vi "Equalizer.vi"() -> ()   [LabVIEW 2018]
uses:
  <vilib>/Analysis/2dsp.llb/Power Spectrum (DBL).vi
  <vilib>/Analysis/NI_AALPro.lvlib
panel:
  in  "False case signal":bool
  in  "Signal":dbl
  in  "Highpass":bool
  in  "Lowpass":bool
  in  "Bandpass":bool
  out "Highpass":bool
  out "Bandpass":bool
  out "Lowpass":bool
  out "Waveform Chart":dbl[](graph)
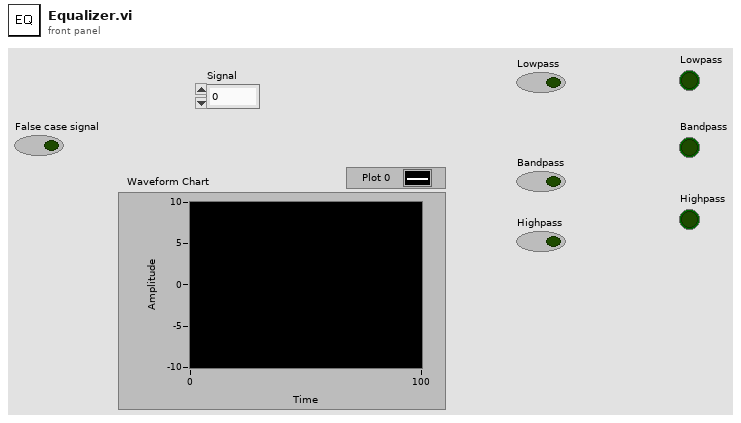
[diagram p1: front panel]
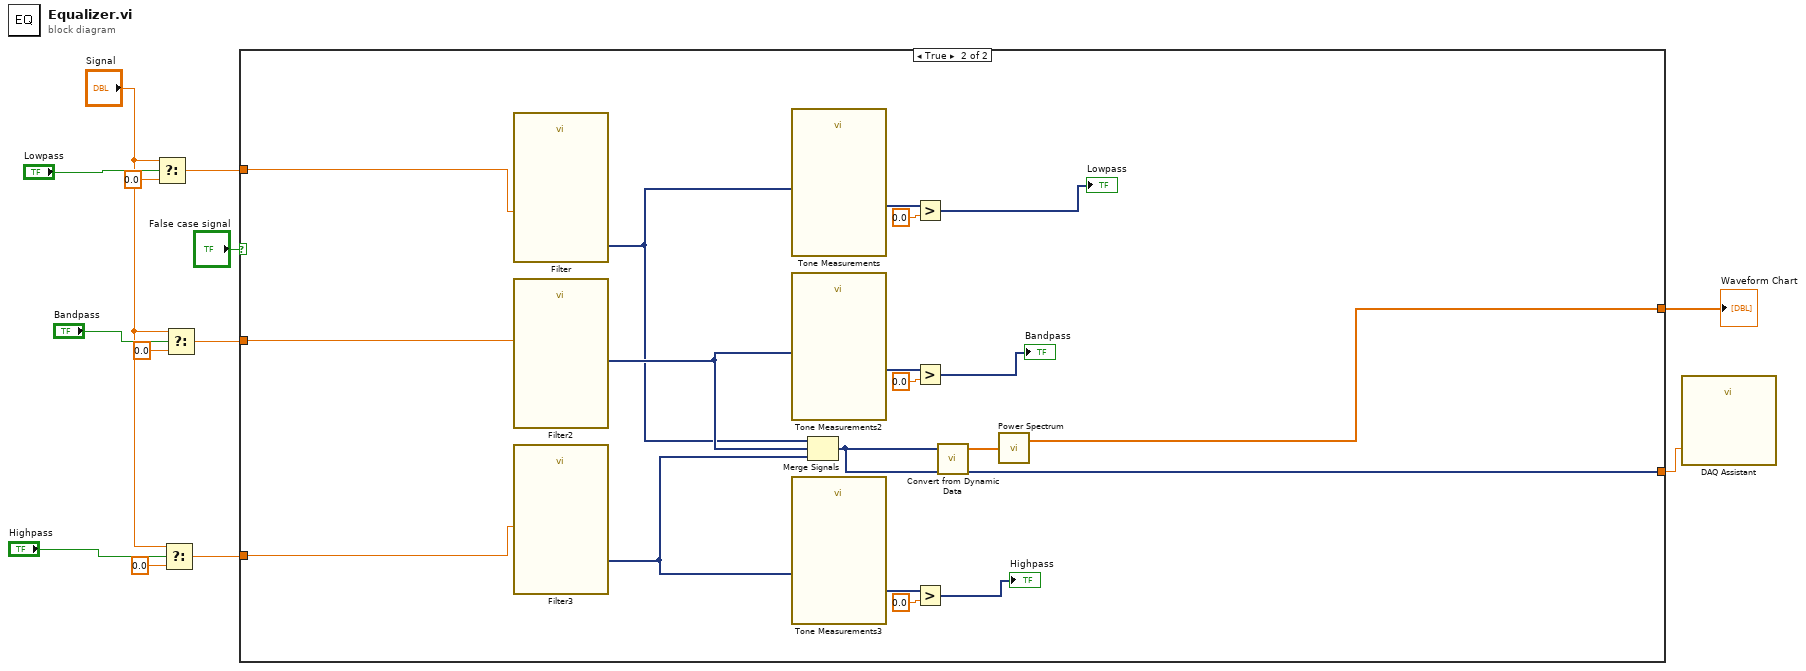
[diagram p0: block diagram]
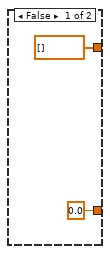
[diagram p2: hidden frame]
diagram:
  n1 = Select(t="Signal", s="Lowpass", f=0.0) -> (s? t:f=w10:dbl)
  n2 = Select(t="Signal", s="Highpass", f=0.0) -> (s? t:f=w8:dbl)
  n3 = Select(t="Signal", s="Bandpass", f=0.0) -> (s? t:f=w9:dbl)
  n4 = case shown="True" "False case signal" {
    tunnel: w10 -> [_ w20]
    tunnel: w9 -> [_ w19]
    tunnel: w8 -> [_ w18]
    tunnel: [0.0 w17] -> w6
    tunnel: [dbl[] [] ("Power Spectrum") w16] -> w5
    frame False {
    }
    frame True {
      n5 = call "Filter"("Signal"=w20) -> ("Filtered Signal"=w28:dynamicdata)  [unwired: 9 in, 1 out]
      n6 = call "Filter2"("Signal"=w19) -> ("Filtered Signal"=w29:dynamicdata)  [unwired: 9 in, 1 out]
      n7 = call "Filter3"("Signal"=w18) -> ("Filtered Signal"=w30:dynamicdata)  [unwired: 9 in, 1 out]
      n8 = call "Tone Measurements"("Signals"=w28) -> ("Amplitude"=w31:dynamicdata)  [unwired: 8 in, 2 out]
      n9 = call "Tone Measurements2"("Signals"=w29) -> ("Amplitude"=w25:dynamicdata)  [unwired: 8 in, 2 out]
      n10 = call "Tone Measurements3"("Signals"=w30) -> ("Amplitude"=w27:dynamicdata)  [unwired: 8 in, 2 out]
      n11 = Merge Signals(w28, w29, w30) -> (w17:dynamicdata)
      n12 = Greater?(x=w31, y=0.0) -> (0:→"Lowpass":dynamicdata)
      n13 = Greater?(x=w25, y=0.0) -> (0:→"Bandpass":dynamicdata)
      n14 = Greater?(x=w27, y=0.0) -> (0:→"Highpass":dynamicdata)
      n15 = call "Convert from Dynamic Data"("Dynamic Data Type"=w17) -> ("Array"=w21:dbl[])  [unwired: 3 in]
      n16 = call-poly <vilib>:"Power Spectrum.vi"("X"=w21) -> ("Power Spectrum"=w16:dbl[])  [unwired: 1 out]
    }
  }
  "Waveform Chart" <- w5
  n17 = call "DAQ Assistant"("data"=w6) -> ()  [unwired: 17 in, 2 out]
